vi "Initialize.vi"(8 "error in (no error)":errorcluster, 11 "TCP in":refnum<class "TCP.lvclass">) -> (0 "error out":errorcluster, 3 "TCP out":refnum<class "TCP.lvclass">)   [LabVIEW 2021, in "TCP.lvclass"]
uses:
  TCP.lvclass
  D:/my_projects/projects/Algorithms/Labview/21/Modbus_v121c/Network Protocol/MB/Modbus Master CR.lvclass
  D:/my_projects/projects/Algorithms/Labview/21/Modbus_v121c/Network Protocol/Network Protocol.lvclass
  MB Param/MBTCP Param/MBTCP Param.lvclass
  MB/ctl/MB timeouts.ctl
  Transmission Data Unit/IP/IP Data Unit.lvclass
  D:/my_projects/projects/Algorithms/Labview/21/Modbus_v121c/Transmission Data Unit/Transmission Data Unit.lvclass
  MB/Modbus Master CR.lvclass/Modbus Master CR.ctl
  MB Param/MBTCP Param/MBTCP Param.lvclass/MBTCP Param.ctl
  Transmission Data Unit/IP/IP Data Unit.lvclass/IP Data Unit.ctl
  Transmission Data Unit/Transmission Data Unit.lvclass/Transmission Data Unit.ctl
  Network Protocol.lvclass/Network Protocol.ctl
  Transmission Data Unit/IP/Write address.vi
  Transmission Data Unit/IP/Write port.vi
  Transmission Data Unit/IP/Write connect timeout.vi
  MB/Modbus Master CR.lvclass
  Transmission Data Unit/Transmission Data Unit.lvclass
  Network Protocol.lvclass
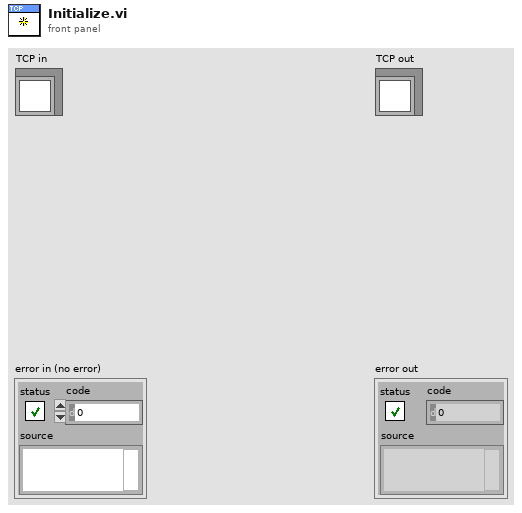
[diagram p1: front panel]
types:
  T1 = typedef "Modbus Master CR.lvclass/MB timeouts.ctl" = cluster{"reconn_timeout":i32, "N attempt max":i32, "t_reset_TTL":i32, "period":i32}
  T2 = typedef "MBParam.lvlib/MBTCP Param.lvclass/timeouts.ctl" = cluster{"conn_timeout":i32, "reconn_timeout":i32, "N attempt max":i32, "t_reset_TTL":i32, "write_timeout":i32, "read_timeout":i32, "period":i32}
  T3 = cluster{"Remote IP Address":string, "Remote Port":u16}
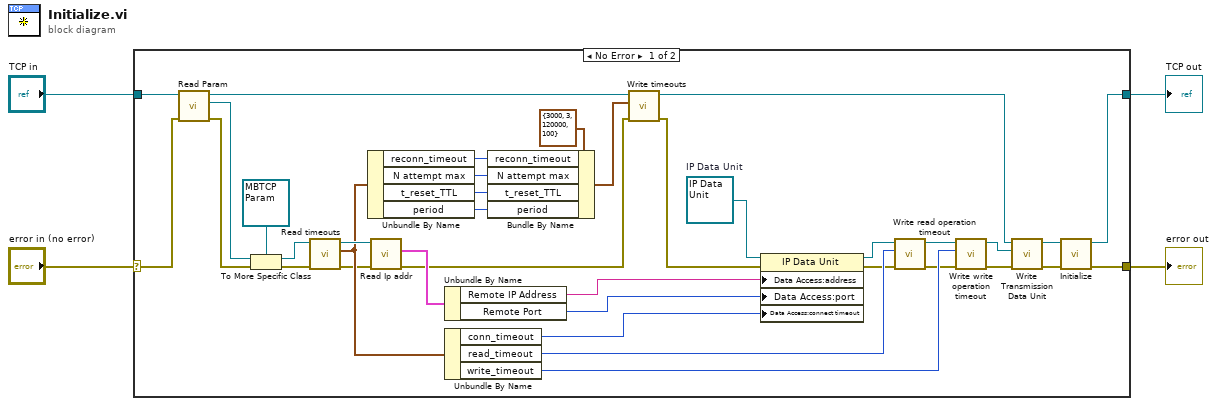
[diagram p0: block diagram]
diagram:
  n1 = case shown="No Error" "error in (no error)" {
    selector: "error in (no error)" -> [w31 w42]
    tunnel: [w18 w42] -> w3
    tunnel: [w19 w43] -> w1
    tunnel: "TCP in" -> [w28 w43]
    frame No Error {
      w17 = refnum<class "IP Data Unit.lvclass"> refnum  # IP Data Unit
      n2 = call "Read Param.vi"("error in (no error)"=w31, "MB_TCP in"=w28) -> ("error out"=w30:errorcluster, "Param"=w27:refnum<class "MB Param.lvclass">, "MB_TCP out"=w26:refnum<class "TCP.lvclass">)  [unwired: 7 in]
      n3 = To More Specific Class(target class=refnum<class "MBTCP Param.lvclass"> refnum ("MBParam.lvlib:MBTCP Param.lvclass"), reference=w27, error in=w30) -> (specific class reference=w29:refnum<class "MBTCP Param.lvclass">, error out=w40:errorcluster)
      n4 = call "Read timeouts.vi"("error in (no error)"=w40, "MBParam in"=w29) -> ("error out"=w21:errorcluster, "timeouts"=w25:T2, "MBParam out"=w33:refnum<class "MBTCP Param.lvclass">)  [unwired: 7 in]
      n5 = Unbundle By Name(w25) -> ("reconn_timeout"=w38:i32, "N attempt max"=w35:i32, "t_reset_TTL"=w36:i32, "period"=w37:i32)
      n6 = call "Read Ip addr.vi"("error in (no error)"=w21, "MBParam in"=w33) -> ("error out"=w20:errorcluster, "IP address"=w32:T3)  [unwired: 7 in, 1 out]
      n7 = Unbundle By Name(w32) -> ("Remote IP Address"=w15:string, "Remote Port"=w14:u16)
      n8 = Unbundle By Name(w25) -> ("conn_timeout"=w13:i32, "read_timeout"=w11:i32, "write_timeout"=w22:i32)
      n9 = Bundle By Name(cluster=T1 {"reconn_timeout"=3000, "N attempt max"=3, "t_reset_TTL"=120000, "period"=100} ("MB timeouts"), "reconn_timeout"=w38, "N attempt max"=w35, "t_reset_TTL"=w36, "period"=w37) -> (w34:T1)
      n10 = call "Write timeouts.vi"("error in (no error)"=w20, "MB timeouts"=w34, "MB_TCP in"=w26) -> ("error out"=w16:errorcluster, "MB_TCP out"=w7:refnum<class "TCP.lvclass">)  [unwired: 7 in]
      n11 = property class="IP Data Unit"(reference=w17, error in=w16, "Data Access:address"=w15, "Data Access:port"=w14, "Data Access:connect timeout"=w13) -> (reference out=w12:refnum<class "IP Data Unit.lvclass">, error out=w10:errorcluster)
      n12 = call "Write read operation timeout.vi"("error in (no error)"=w10, "read operation timeout"=w11, "transmission data unit in"=w12) -> ("error out"=w9:errorcluster, "transmission data unit out"=w8:refnum<class "IP Data Unit.lvclass">)  [unwired: 7 in]
      n13 = call "Write write operation timeout.vi"("error in (no error)"=w9, "write operation timeout"=w22, "transmission data unit in"=w8) -> ("error out"=w24:errorcluster, "transmission data unit out"=w23:refnum<class "IP Data Unit.lvclass">)  [unwired: 7 in]
      n14 = call "Write Transmission Data Unit.vi"("error in (no error)"=w24, "Transmission Data Unit"=w23, "Network Protocol in"=w7) -> ("error out"=w5:errorcluster, "Network Protocol out"=w6:refnum<class "TCP.lvclass">)  [unwired: 7 in]
      n15 = call-parent "Initialize.vi"("error in (no error)"=w5, "MB in"=w6) -> ("error out"=w18:errorcluster, "MB out"=w19:refnum<class "TCP.lvclass">)  [unwired: 8 in]
    }
    frame Error {
    }
  }
  "error out" <- w3
  "TCP out" <- w1
